vi "Register Event.vi"(4 "Get Last Broadcast Event (F)":bool, 6 "Event Handler":refnum<class "Abstract Event Message for View.lvclass">, 7 "Event":refnum<class "Event.lvclass">, 8 "error in (no error)":errorcluster, 11 "View in":refnum<class "View.lvclass">) -> (0 "error out":errorcluster, 3 "View out":refnum<class "View.lvclass">)   [LabVIEW 2023, in "MVC Actors.lvlib" / "View.lvclass"]
doc: "Registers an event to the Controller by specifying the concrete event and the corresponding Event Handler. If \"Get Last Broadcast Event (F)\" is TRUE the View will receive the last broadcast Event."
uses:
  View.lvclass
  Event Handlers/Abstract Event Message for View/Abstract Event Message for View.lvclass
  Event/Event.lvclass
  View.lvclass/View.ctl
  properties/Read Controller Actor Enqueuer.vi
  properties/Read Name.vi
  <vilib>/ActorFramework/Message Enqueuer/Message Enqueuer.lvclass
  Controller Messages/Register by Name Msg/Register by Name Msg.lvclass
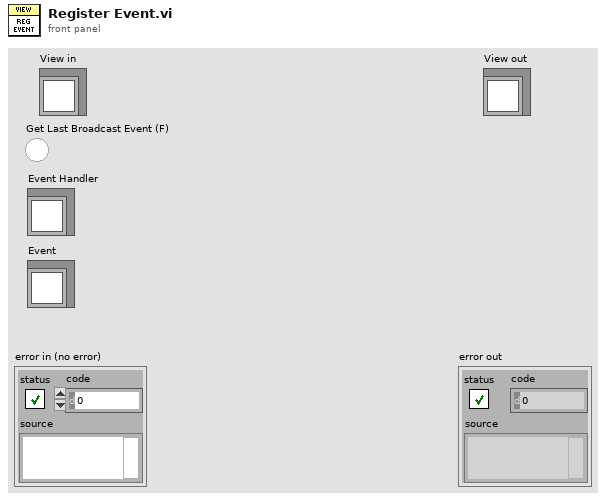
[diagram p1: front panel]
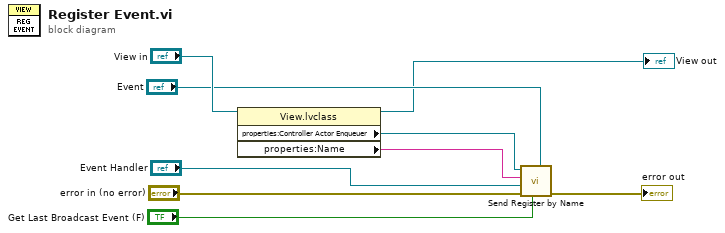
[diagram p0: block diagram]
diagram:
  n1 = property class="View.lvclass"(reference="View in") -> (reference out=→"View out":refnum<class "View.lvclass">, "properties:Controller Actor Enqueuer"=w4:refnum<class "Message Enqueuer.lvclass">, "properties:Name"=w5:string)  [unwired: 1 in, 1 out]
  n2 = call "Send Register by Name.vi"("Event"="Event", "Get Last Broadcast Event (F)"="Get Last Broadcast Event (F)", "error in (no error)"="error in (no error)", "Event Fire Handler"="Event Handler", "View Name"=w5, "Message Enqueuer in"=w4) -> ("error out"=→"error out":errorcluster)  [unwired: 4 in, 1 out]
